vi "Read Phase (cycles).vi"(8 "error in (no error)":errorcluster, 11 "Tone in":refnum<class "Tone.lvclass">) -> (0 "error out":errorcluster, 2 "Phase (cycles)":dbl, 3 "Tone out":refnum<class "Tone.lvclass">)   [LabVIEW 2020, in "Tone.lvclass"]
uses:
  Tone.lvclass
  Tone.lvclass/Tone.ctl
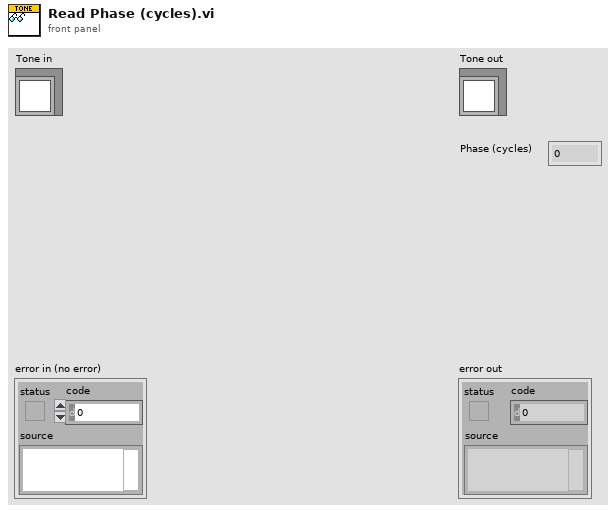
[diagram p1: front panel]
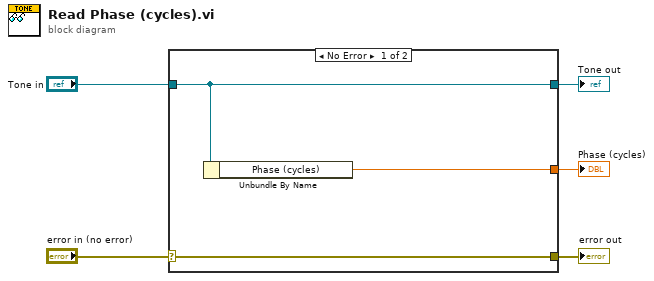
[diagram p0: block diagram]
diagram:
  n1 = case shown="No Error" "error in (no error)" {
    selector: "error in (no error)" -> [w8 w9]
    tunnel: [w8 w9] -> w4
    tunnel: [w7 w10] -> w2
    tunnel: "Tone in" -> [w7 w10]
    tunnel: [w6 _] -> w1
    frame No Error {
      n2 = Unbundle By Name(w7) -> ("Phase (cycles)"=w6:dbl)
    }
    frame Error {
    }
  }
  "error out" <- w4
  "Tone out" <- w2
  "Phase (cycles)" <- w1
